vi "Init Camera.vi"(7 "Trigger Jitter (ms)":dbl, 8 "error in (no error)":errorcluster, 10 "Physical Camera Assignment":T1[](array[typedef]), 11 "Hamamatsu Camera in":refnum<class "Hamamatsu Camera.lvclass">) -> (0 "error out":errorcluster, 2 "Installed Cameras":T1[](array[typedef]), 3 "Hamamatsu Camera out":refnum<class "Hamamatsu Camera.lvclass">)   [LabVIEW 2023, in "Hamamatsu Camera.lvlib" / "Hamamatsu Camera.lvclass"]
uses:
  Hamamatsu Camera.lvclass
  Resources/Type Defs/Physical Camera Assignment.ctl
  Hamamatsu Camera.lvclass/Hamamatsu Camera.ctl
  Camera/Camera.lvclass
  Hamamatsu Camera.lvlib
panel:
  out "Model":string
  out "Camera Details":T2(array[cluster])
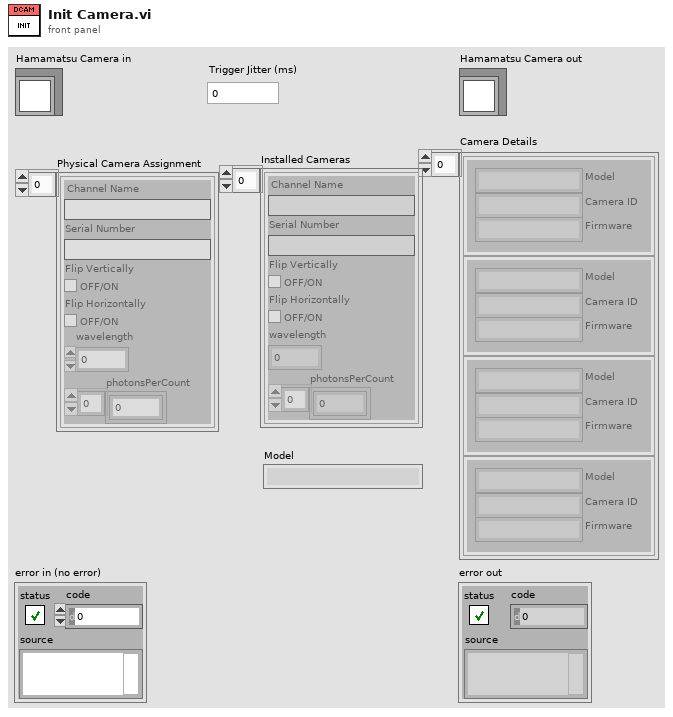
[diagram p1: front panel]
types:
  T1 = typedef "Physical Camera Assignment.ctl" = cluster{"Channel Name":string, "Serial Number":string, "Flip Vertically":bool, "Flip Horizontally":bool, "wavelength":i16, "photonsPerCount":dbl[]}
  T2 = cluster{"Model":string, "Camera ID":string, "Firmware":string}[]
  T3 = typedef "LVMinMaxIncTypeDef.ctl" = cluster{"Minimum":dbl, "Maximum":dbl, "Increment":dbl}
  T4 = cluster{"H Offset":cluster{"Value":i32, "Limits":T3}, "V Offset":cluster{"Value":i32, "Limits":T3}, "H Size":cluster{"Value":i32, "Limits":T3}, "V Size":cluster{"Value":i32, "Limits":T3}}
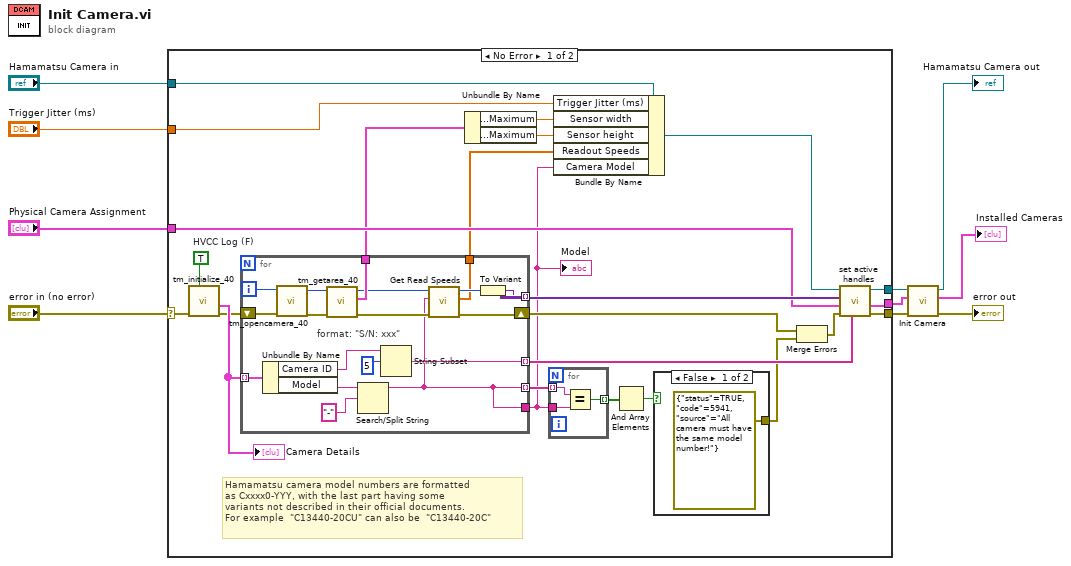
[diagram p0: block diagram]
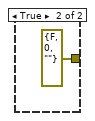
[diagram p2: hidden frame]
diagram:
  n1 = case shown="No Error" "error in (no error)" {
    selector: "error in (no error)" -> [w33 w60]
    tunnel: [w27 w60] -> w5
    tunnel: "Hamamatsu Camera in" -> [w18 w59]
    tunnel: [w19 w59] -> w6
    tunnel: "Physical Camera Assignment" -> [w28 w58]
    tunnel: [w26 w58] -> w3
    tunnel: "Trigger Jitter (ms)" -> [w16 _]
    frame No Error {
      w32 = TRUE  # HVCC Log (F)
      # "Hamamatsu camera model numbers are formatted\nas Cxxxx0-YYY, with the last part having some\nvariants not described in their official documents.\nFor example  \"C13440-20CU\" can also be  \"C13440-20C\""
      n2 = call <userlib>:"tm_initialize_40.vi"("HVCC Log (F)"=w32, "error in (no error)"=w33) -> ("error out"=w31:errorcluster, "Camera Details Array"=w34:T2)  [unwired: 6 in, 2 out]
      "Camera Details" <- w34
      n3 = for {
        tunnel: w34 -> [w52] mode=indexing
        tunnel: [w35] -> w25 mode=indexing
        tunnel: [w49] -> w30 mode=indexing
        shift-right: [w37] -> w21
        shift-left: w31 -> [w47]
        tunnel: [w46] -> w29 mode=indexing
        tunnel: [w35] -> w12
        tunnel: [w41] -> w15
        tunnel: [w36] -> w11
        i -> [w48]
        # "format: \"S/N: xxx\""
        n4 = Unbundle By Name(w52) -> ("Camera ID"=w50:string, "Model"=w45:string)
        n5 = call <userlib>:"tm_opencamera_40.vi"("error in (no error)"=w47, "Camera Index"=w48) -> ("error out"=w43:errorcluster, "Handle out"=w42:u32)  [unwired: 7 in, 1 out]
        n6 = call <userlib>:"tm_getarea_40.vi"("error in (no error)"=w43, "Handle in"=w42) -> ("error out"=w40:errorcluster, "Sub Region"=w41:T4, "Handle out"=w39:u32)  [unwired: 7 in]
        n7 = Search/Split String(string=w45, search string/char (-)="-") -> (substring before match=w35:string)  [unwired: 1 in, 2 out]
        n8 = String Subset(string=w50, offset (0)=5) -> (substring=w49:string)  [unwired: 1 in]
        n9 = call "Get Read Speeds.vi"("error in (no error)"=w40, "camera model"=w35, "Handle in"=w39) -> ("error out"=w37:errorcluster, "Readout Speeds"=w36:dbl[], "Handle out"=w38:u32)  [unwired: 6 in]
        n10 = To Variant(anything=w38) -> (Variant=w46:variant)
      }
      "Model" <- w12
      n11 = Unbundle By Name(w15) -> ("H Size.Limits.Maximum"=w14:dbl, "V Size.Limits.Maximum"=w13:dbl)
      n12 = for {
        tunnel: w12 -> [w57]
        tunnel: w25 -> [w56] mode=indexing
        tunnel: [w55] -> w24 mode=indexing
        n13 = Equal?(x=w56, y=w57) -> (x = y?=w55:bool)
      }
      n14 = Bundle By Name(cluster=w18, "Trigger Jitter (ms)"=w16, "Sensor width"=w14, "Sensor height"=w13, "Readout Speeds"=w11, "Camera Model"=w12) -> (w17:refnum<class "Hamamatsu Camera.lvclass">)
      n15 = And Array Elements(Boolean array=w24) -> (logical AND=w23:bool)
      n16 = case shown="False" w23 {
        tunnel: [errorcluster {"status"=TRUE, "code"=5941, "source"="All camera must have the same model number!"} ("error constant") errorcluster {"status"=FALSE, "code"=0, "source"=""} ("error constant")] -> w20
        frame False {
        }
        frame True {
        }
      }
      n17 = Merge Errors(w21, w20) -> (w22:errorcluster)
      n18 = call-dynamic "set active handles.vi"("serial numbers"=w30, "error in (no error)"=w22, "All Camera"=w28, "All Handles"=w29, "Camera in"=w17) -> ("error out"=w27:errorcluster, "Selected cameras"=w26:T1[], "Camera out"=w19:refnum<class "Hamamatsu Camera.lvclass">)  [unwired: 3 in, 1 out]
    }
    frame Error {
    }
  }
  n19 = call-parent "Init Camera.vi"("error in (no error)"=w5, "Physical Camera Assignment"=w3, "Camera in"=w6) -> ("error out"=→"error out":errorcluster, "Installed Cameras"=→"Installed Cameras":T1[], "Camera out"=→"Hamamatsu Camera out":refnum<class "Hamamatsu Camera.lvclass">)  [unwired: 6 in]
